vi "FGV_REWORK_DIAGNOSTICS_single_message_display.vi"(4 "front_panel_reference":refnum<vi>, 6 "SQL_listbox_reference":refnum<vi>, 7 "options":T1, 8 "error_in":errorcluster, 11 "input":variant) -> (0 "error_out":errorcluster)   [LabVIEW 2019]
uses:
  FGV_REWORK_DIAGNOSTICS_single_message_display.ctl
  _misc/AULocalize/SubVIs/Get Localized Phrase Compact Interface 1D.vi
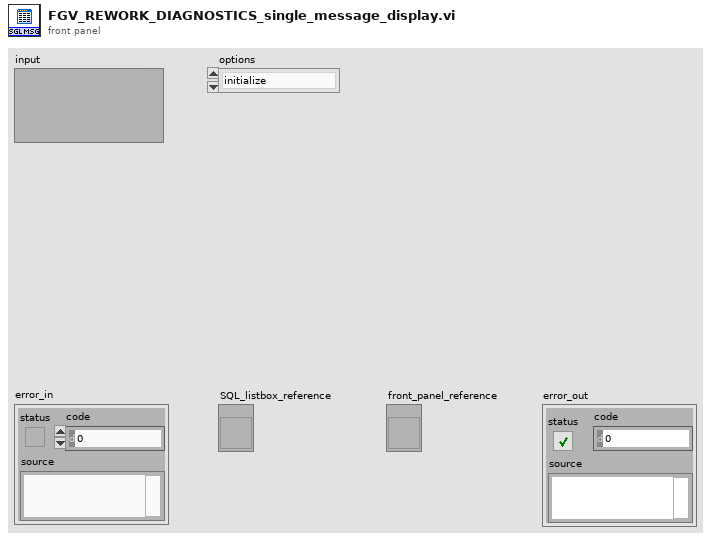
[diagram p1: front panel]
types:
  T1 = typedef "FGV_REWORK_DIAGNOSTICS_single_message_display.ctl" = enum16{"initialize", "display_message"}
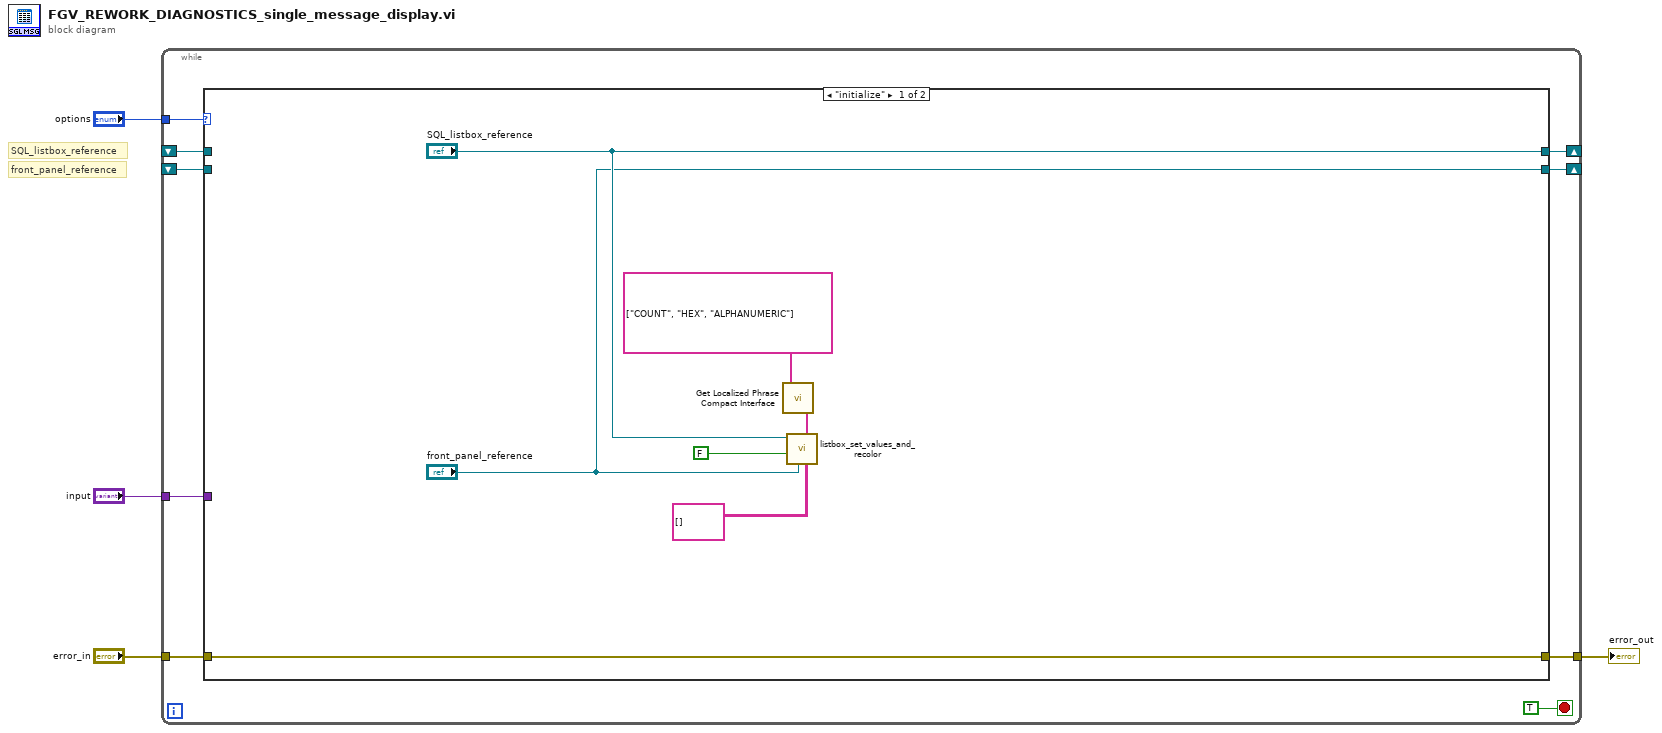
[diagram p0: block diagram]
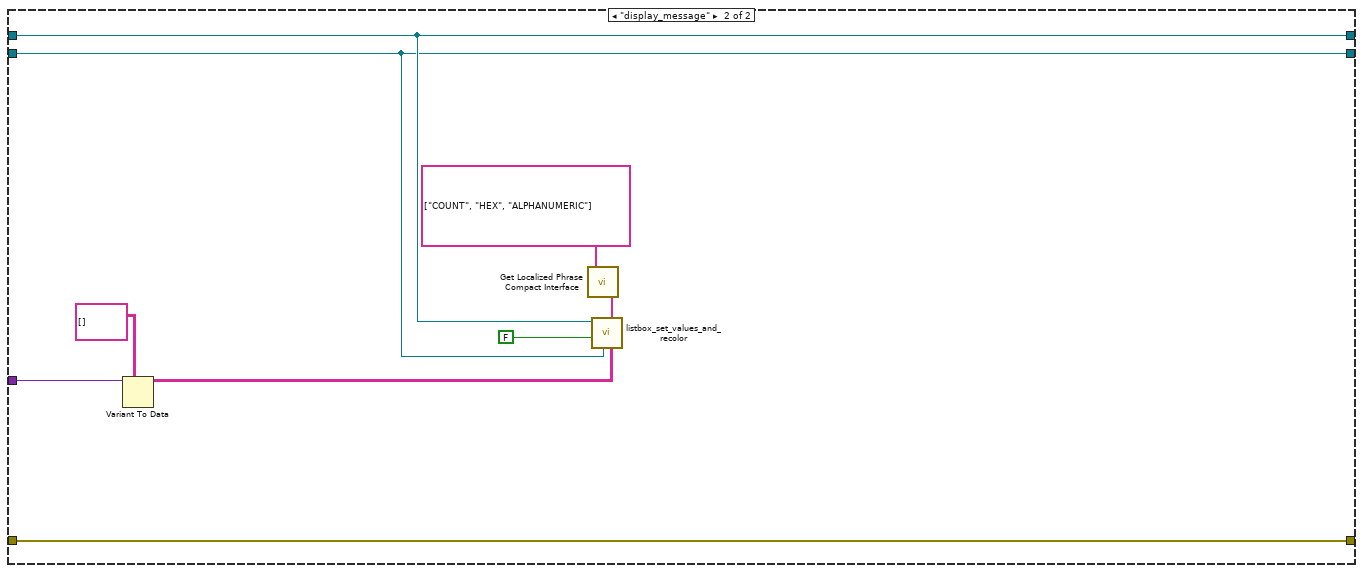
[diagram p2: hidden frame]
diagram:
  # "front_panel_reference"
  # "SQL_listbox_reference"
  n1 = while {
    tunnel: "options" -> [w12]
    tunnel: [w11] -> w4
    tunnel: "error_in" -> [w10]
    shift-right: [w9] -> _
    shift-left: _ -> [w8]
    tunnel: "input" -> [w7]
    shift-right: [w6] -> _
    shift-left: _ -> [w5]
    stop <- TRUE stop-if-true
    n2 = case shown="\"initialize\"" w12 {
      tunnel: [w20 w29] -> w11
      tunnel: w10 -> [w20 w29]
      tunnel: ["SQL_listbox_reference" w26] -> w9
      tunnel: w8 -> [_ w26]
      tunnel: w7 -> [_ w24]
      tunnel: ["front_panel_reference" w25] -> w6
      tunnel: w5 -> [_ w25]
      frame "initialize" {
        n3 = call-poly "Get Localized Phrase Compact Interface.vi"("Key"=string[] ["COUNT", "HEX", "ALPHANUMERIC"] ("column_names")) -> ("Translated Phrase"=w14:string[])
        n4 = call "listbox_set_values_and_recolor.vi"("item_names"=string[][] [], "front_panel_reference"="front_panel_reference", "column_names"=w14, "Autosize? (T)"=FALSE, "multicolumn_listbox_reference_in"="SQL_listbox_reference") -> ()  [unwired: 5 in, 2 out]
      }
      frame "display_message" {
        n5 = Variant To Data(type=string[][] [] ("item_names"), Variant=w24) -> (data=w22:string[][])  [unwired: 1 in, 1 out]
        n6 = call-poly "Get Localized Phrase Compact Interface.vi"("Key"=string[] ["COUNT", "HEX", "ALPHANUMERIC"] ("column_names")) -> ("Translated Phrase"=w21:string[])
        n7 = call "listbox_set_values_and_recolor.vi"("item_names"=w22, "front_panel_reference"=w25, "column_names"=w21, "Autosize? (T)"=FALSE, "multicolumn_listbox_reference_in"=w26) -> ()  [unwired: 5 in, 2 out]
      }
    }
  }
  "error_out" <- w4
